vi "Update Timer Data (GPD and Stim).vi"(5 "Timer Data In in":T1) -> (1 "Interval Up?":bool, 2 "Timer Data In out":T1)   [LabVIEW 2019]
uses:
  Controls/Timer Data.ctl
  Lee Lab/CP FES Walking 2018/Code/Working/LabVIEW/Controls/States/Stim Timer State.ctl
  Controls/Protocol Interval.ctl
  Controls/Stim Interval Mode.ctl
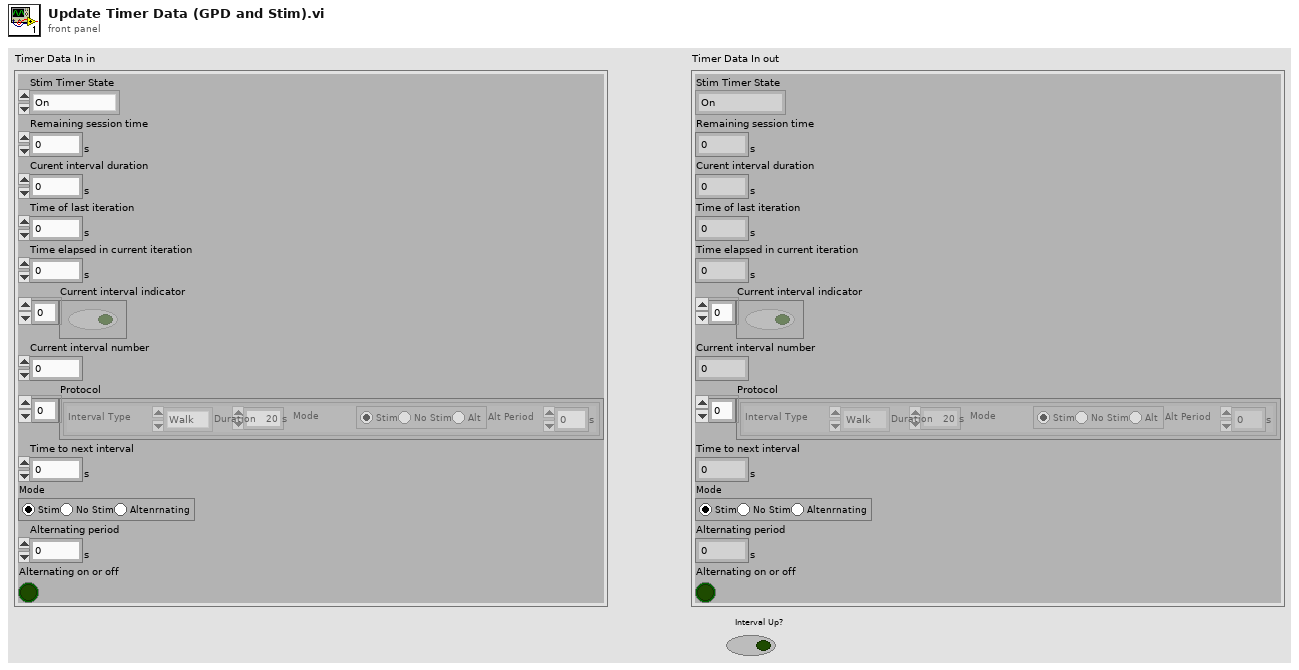
[diagram p1: front panel]
types:
  T1 = typedef "Timer Data.ctl" = cluster{"Stim Timer State":T2, "Remaining session time":dbl[unit], "Curent interval duration":dbl[unit], "Time of last iteration":dbl[unit], "Time elapsed in current iteration":dbl[unit], "Current interval indicator":bool[], "Current interval number":u32, "Protocol":T3[], "Time to next interval":dbl[unit], "Mode":T4, "Alternating period":dbl[unit], "Alternating on or off":bool}
  T2 = typedef "Stim Timer State.ctl" = enum16{"On", "Off", "Initialize", "Stop", "Alternating", "Pause", "Start Timer", "Reset Timer"}
  T3 = typedef "Protocol Interval.ctl" = cluster{"Interval Type":enum16{"Walk", "Rest"}, "Duration":dbl[unit], " Mode":T4, "Alt Period":dbl[unit]}
  T4 = typedef "Stim Interval Mode.ctl" = enum32{"Stim", "No Stim", "Alternating"}
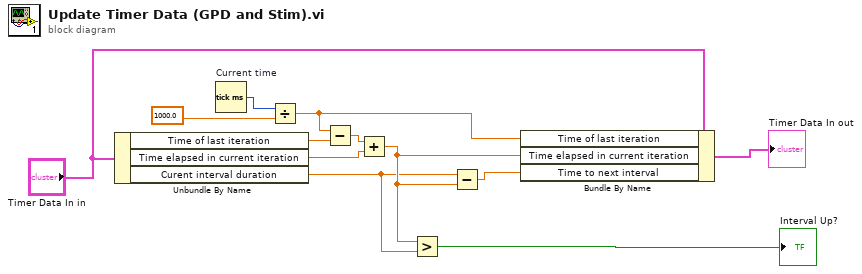
[diagram p0: block diagram]
diagram:
  n1 = Unbundle By Name("Timer Data In in") -> ("Time of last iteration"=w5:dbl[unit], "Time elapsed in current iteration"=w4:dbl[unit], "Curent interval duration"=w8:dbl[unit])
  n2 = Tick Count (ms) "Current time"() -> (millisecond timer value=w3:u32)
  n3 = Divide(x=w3, y=dbl[unit] 1000.0 ("Time of last iteration")) -> (x/y=w1:dbl[unit])
  n4 = Subtract(x=w1, y=w5) -> (x-y=w6:dbl[unit])
  n5 = Add(x=w6, y=w4) -> (x+y=w9:dbl[unit])
  n6 = Greater?(x=w9, y=w8) -> (0:→"Interval Up?":bool)
  n7 = Subtract(x=w8, y=w9) -> (x-y=w10:dbl[unit])
  n8 = Bundle By Name(cluster="Timer Data In in", "Time of last iteration"=w1, "Time elapsed in current iteration"=w9, "Time to next interval"=w10) -> (→"Timer Data In out":T1)
